vi "uObserver_Set_Policy_Sub.vi"(8 "error in (no error)":errorcluster, 10 "uPolicy":refnum<class "uPolicy.lvclass">, 11 "uObserver in":refnum<class "uObserver.lvclass">) -> (0 "error out":errorcluster, 3 "uObserver out":refnum<class "uObserver.lvclass">)   [LabVIEW 2021, in "uFramework_pack_uActor.lvlib" / "uObserver.lvclass"]
doc: "Set the subscription policy: An external caller may pass in the subscription policy to the callee prior to launching it, OR most typically the observer actor itself may internally have its subscription policy either statically defined by the class' Registration override method, or instead of static definition it might take the policy provided by the caller and update it prior to executing the registration action."
uses:
  uObserver.lvclass
  Bin/uFramework.lvlibp/uPolicy/uPolicy.lvclass
  uObserver.lvclass/uObserver.ctl
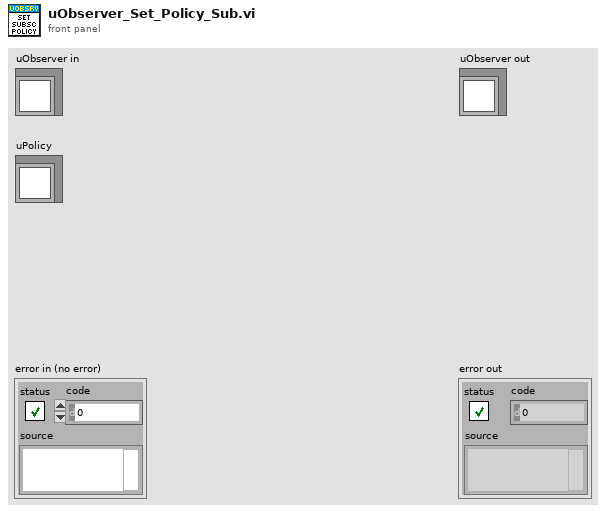
[diagram p1: front panel]
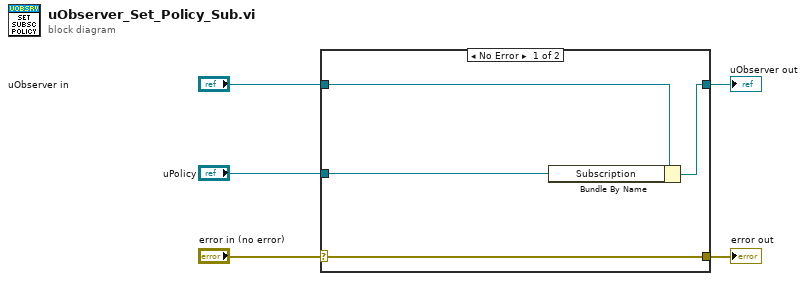
[diagram p0: block diagram]
diagram:
  n1 = case shown="No Error" "error in (no error)" {
    selector: "error in (no error)" -> [w9 w10]
    tunnel: [w9 w10] -> w4
    tunnel: [w7 w11] -> w2
    tunnel: "uObserver in" -> [w8 w11]
    tunnel: "uPolicy" -> [w6 _]
    frame No Error {
      n2 = Bundle By Name(cluster=w8, "Subscription"=w6) -> (w7:refnum<class "uObserver.lvclass">)
    }
    frame Error {
    }
  }
  "error out" <- w4
  "uObserver out" <- w2
